vi "RD Digital Uart Tx.vi"(8 "error in (no error)":errorcluster caption="错误输入（无错误）", 9 "length":i32, 10 "data":u8[](array[numeric]), 11 "handle":u64) -> (0 "error out":errorcluster caption="错误输出", 1 "function return":i32, 3 "handle out":u64)   [LabVIEW 2018, in "InstrumentsPlayground.lvlib"]
doc: "CLIFFAPI int CliffDigitalUartRateSet(FT_HANDLE handle, double rate); CLIFFAPI int CliffDigitalUartRxSet(FT_HANDLE handle, int dio); CLIFFAPI int CliffDigitalUartBitsSet(FT_HANDLE handle, int bits); CLIFFAPI int CliffDigitalUartParitySet(FT_HANDLE handle, int parity); CLIFFAPI int CliffDigitalUartStopSet(FT_HANDLE handle, double stop); CLIFFAPI int CliffDigitalUartTx(FT_HANDLE handle, uchar* data, int length);"
uses:
  InstrumentsPlayground.lvlib
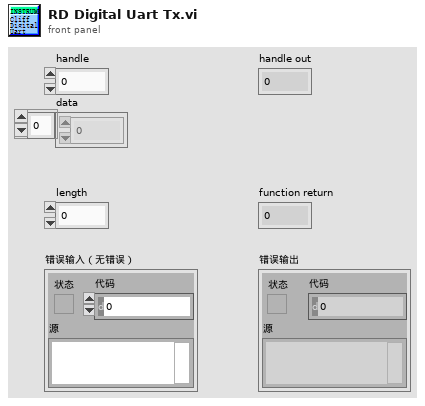
[diagram p1: front panel]
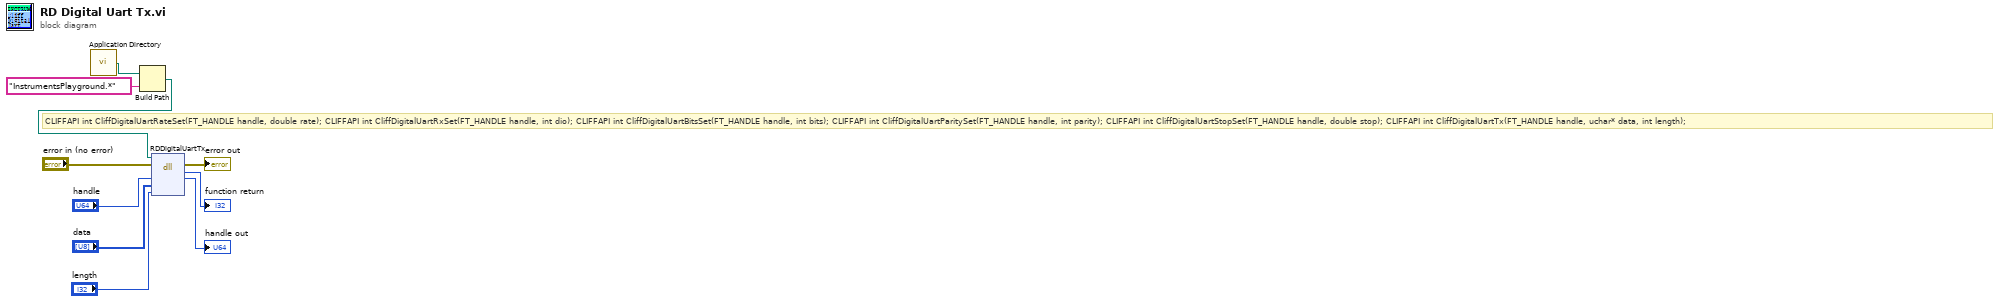
[diagram p0: block diagram]
diagram:
  # "CLIFFAPI int CliffDigitalUartRateSet(FT_HANDLE handle, double rate); CLIFFAPI int CliffDigitalUartRxSet(FT_HANDLE handle, int dio); CLIFFAPI int CliffDigitalUartBitsSet(FT_HANDLE handle, int bits); CLIFFAPI int CliffDigitalUartParitySet(FT_HANDLE handle, int parity); CLIFFAPI int CliffDigitalUartStopSet(FT_HANDLE handle, double stop); CLIFFAPI int CliffDigitalUartTx(FT_HANDLE handle, uchar* data, int length);"
  n1 = call <vilib>:"Application Directory.vi"() -> ("Application Directory"=w3:path)
  n2 = Build Path(base path=w3, name or relative path="InstrumentsPlayground.*" ("名称或相对路径")) -> (appended path=w2:path)
  n3 = dll-call lib="E:/work/YZCourse_Xtext/Cliff/API/LabVIEW lib/InstrumentsPlayground.*" fn="RDDigitalUartTx"(path in=w2, error in="error in (no error)", "handle"="handle", "data"="data", "length"="length") -> (error out=→"error out":errorcluster, "返回类型"=→"function return":i32, "handle"=→"handle out":u64)  [unwired: 3 in, 1 out]
